vi "sub_checkGameResult.vi"(4 "computer symbol":string, 6 "player symbol":string, 11 "control references":refnum<vi>[](array[refnum])) -> (3 "game result":T1)   [LabVIEW 2018]
uses:
  gameStatus.ctl
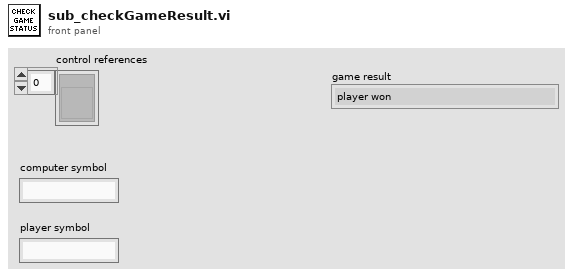
[diagram p1: front panel]
types:
  T1 = typedef "gameStatus.ctl" = enum16{"player won", "computer won", "draw", "no result"}
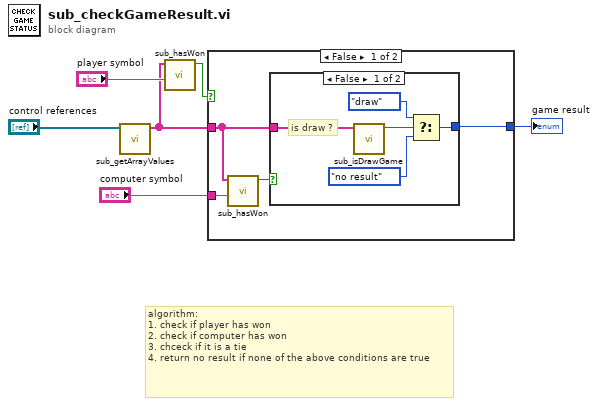
[diagram p0: block diagram]
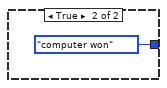
[diagram p2: hidden frame]
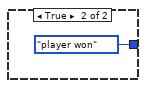
[diagram p3: hidden frame]
diagram:
  # "algorithm: \n1. check if player has won\n2. check if computer has won\n3. chceck if it is a tie\n4. return no result if none of the above conditions are true"
  n1 = call "sub_getArrayValues.vi"("controls"="control references") -> ("array"=w2:string[])  [unwired: 10 in]
  n2 = call "sub_hasWon.vi"("player"="player symbol", "array"=w2) -> ("has won ?"=w4:bool)  [unwired: 9 in]
  n3 = case shown="False" w4 {
    tunnel: [w8 gameStatus."player won" ("game result")] -> w3
    tunnel: w2 -> [w7 _]
    tunnel: "computer symbol" -> [w10 _]
    frame False {
      n4 = call "sub_hasWon.vi"("player"=w10, "array"=w7) -> ("has won ?"=w9:bool)  [unwired: 9 in]
      n5 = case shown="False" w9 {
        tunnel: [w11 gameStatus."computer won" ("game result")] -> w8
        tunnel: w7 -> [w15 _]
        frame False {
          # "is draw ?"
          n6 = call "sub_isDrawGame.vi"("array"=w15) -> ("is draw"=w14:bool)  [unwired: 10 in]
          n7 = Select(t=gameStatus."draw" ("game result"), s=w14, f=gameStatus."no result" ("game result")) -> (s? t:f=w11:T1)
        }
        frame True {
        }
      }
    }
    frame True {
    }
  }
  "game result" <- w3
